vi "Update OOB gRPC Port.vi"(7 "OOB gRPC Port Ref in":refnum<vi>, 8 "error in (no error)":errorcluster) -> (0 "error out":errorcluster)   [LabVIEW 2025, in "I2C Bus Monitor UI.lvlib"]
uses:
  I2C Bus Monitor UI.lvlib
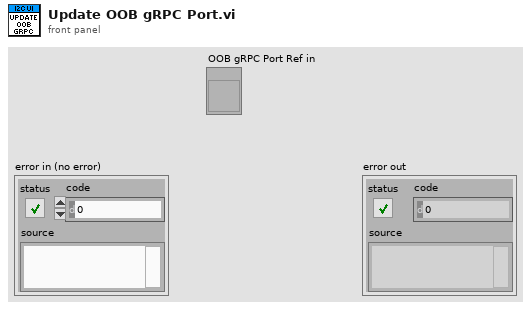
[diagram p1: front panel]
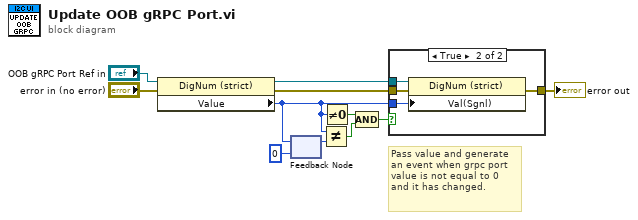
[diagram p0: block diagram]
diagram:
  # "Pass value and generate an event when grpc port value is not equal to 0 and it has changed."
  n1 = property on="Property Node" class="DigNum (strict)"(reference="OOB gRPC Port Ref in", error in="error in (no error)") -> (reference out=w11:refnum<vi>, error out=w2:errorcluster, "Value"=w10:i32)
  n2 = feedback #1(0 ("OOB gRPC Port")) -> (w8:i32)
  n3 = feedback-in #1(w10) -> ()
  n4 = Not Equal?(x=w10, y=w8) -> (x != y?=w7:bool)
  n5 = Not Equal To 0?(x=w10) -> (x != 0?=w5:bool)
  n6 = Compound Arithmetic op=AND(w5, w7) -> (w6:bool)
  n7 = case shown="True" w6 {
    tunnel: w10 -> [_ w16]
    tunnel: w11 -> [_ w15]
    tunnel: w2 -> [w12 w14]
    tunnel: [w12 w13] -> w1
    frame False {
    }
    frame True {
      n8 = property on="Property Node" class="DigNum (strict)"(reference=w15, error in=w14, "Val(Sgnl)"=w16) -> (error out=w13:errorcluster)  [unwired: 1 out]
    }
  }
  "error out" <- w1
